vi "Light_Control_CMD (SubVI).vi"(0 "Front Light Mode":enum8{"Close", "Open", "BLN", "Customize"}(ring), 5 "Front Customize Light (0-100)":u8, 7 "Rear Light Mode":enum8{"Close", "Open", "BLN", "Customize"}(ring), 9 "Rear Customize Light (0-100)":u8, 11 "Frame ID":u8) -> (6 "CMD":u8[](array[numeric]))   [LabVIEW 2019]
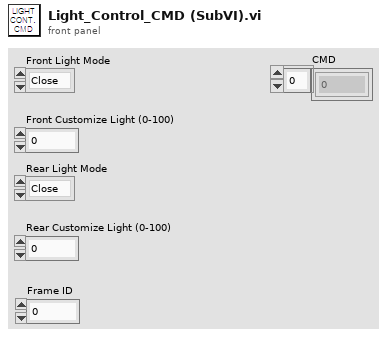
[diagram p1: front panel]
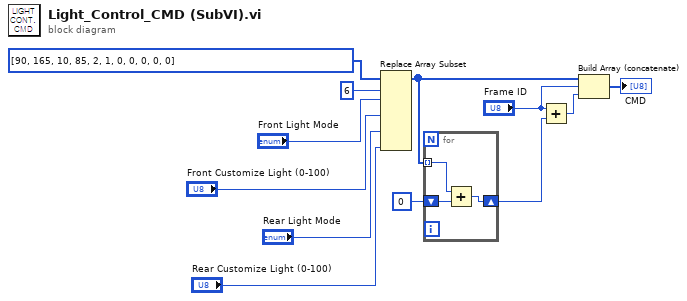
[diagram p0: block diagram]
diagram:
  n1 = Replace Array Subset(array=u8[] [90, 165, 10, 85, 2, 1, 0, 0, 0, 0, 0] ("unsigned byte array"), new element #1="Front Light Mode", index #1=6 ("index"), new element #2="Front Customize Light (0-100)", new element #3="Rear Light Mode", new element #4="Rear Customize Light (0-100)") -> (w8:u8[])  [unwired: 3 in]
  n2 = for {
    tunnel: w8 -> [w15] mode=indexing
    shift-right: [w13] -> w3
    shift-left: u8 0 -> [w14]
    n3 = Add(x=w15, y=w14) -> (x+y=w13:u8)
  }
  n4 = Add(x="Frame ID", y=w3) -> (x+y=w1:u8)
  n5 = Build Array (concatenate)(w8, "Frame ID", w1) -> (→"CMD":u8[])
